vi "蝴蝶图.vi"() -> ()   [LabVIEW 2023]
panel:
  out "XY Graph":cluster{"Y":dbl[], "Y":dbl[]}[](graph)
  out "return value":dbl[][](array[numeric])
  in  "Array 3":dbl[][](array[numeric])
  in  "module path 2":path
  out "error out 2":errorcluster
  out "error out":errorcluster
  in  "module path":path
  out "Array 2":string[](array[string])
  in  "String":string
  in  "Array":string[](array[string])
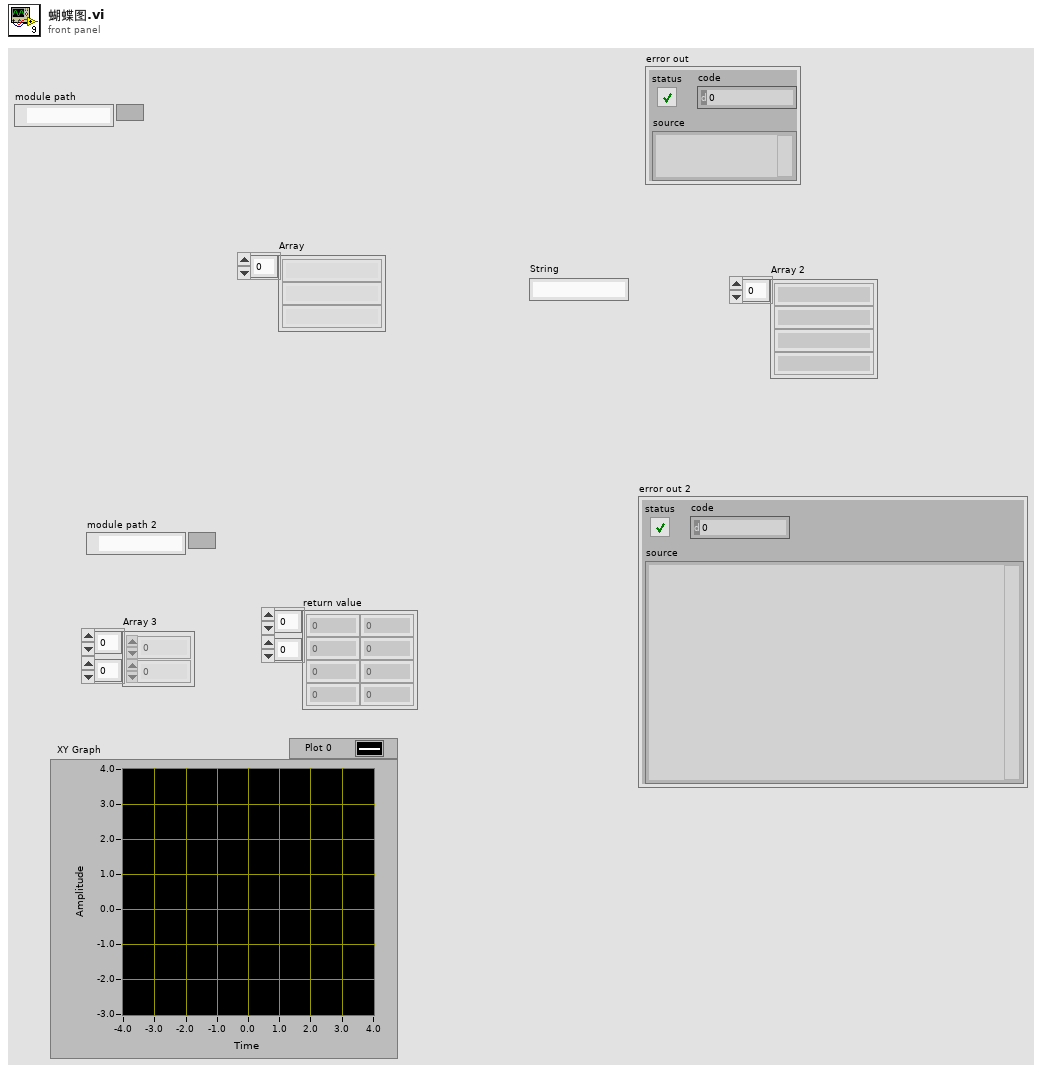
[diagram p1: front panel]
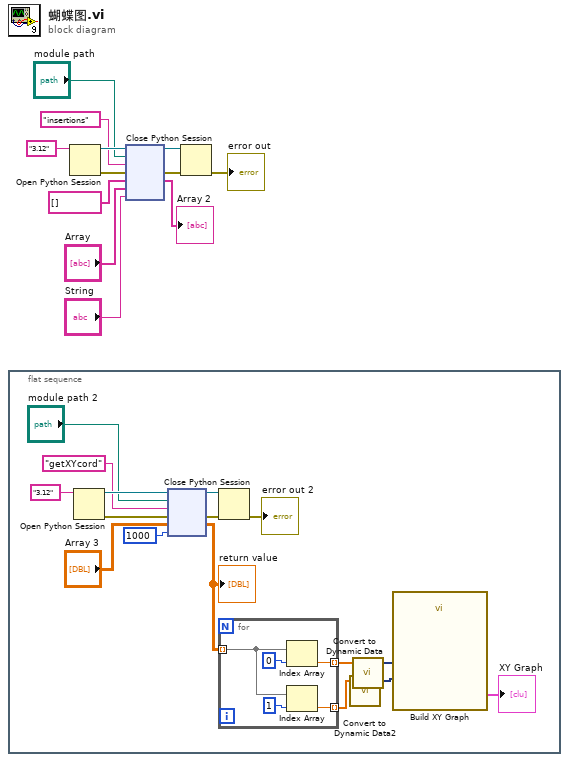
[diagram p0: block diagram]
diagram:
  n1 = flat-sequence {
    frame #0 {
      n2 = Open Python Session(python version="3.12" ("Python version")) -> (session out=w28:refnum<k35>, error out=w26:errorcluster)  [unwired: 2 in]
      n3 = node(w28, "module path 2", "getXYcord" ("function name"), w26, "Array 3", 1000) -> (w27:refnum<k35>, w25:errorcluster, w18:dbl[][])  [unwired: 1 in, 2 out]
      "return value" <- w18
      n4 = Close Python Session(session in=w27, error in=w25) -> (11:→"error out 2":errorcluster)
      n5 = for {
        tunnel: w18 -> [w32] mode=indexing
        tunnel: [w30] -> w16 mode=indexing
        tunnel: [w29] -> w14 mode=indexing
        n6 = Index Array(array=w32, index=0) -> (element=w30:dbl)
        n7 = Index Array(array=w32, index=1) -> (element=w29:dbl)
      }
      n8 = call "Convert to Dynamic Data2"("Array"=w14) -> ("Dynamic Data Type"=w13:dynamicdata)  [unwired: 3 in]
      n9 = call "Convert to Dynamic Data"("Array"=w16) -> ("Dynamic Data Type"=w15:dynamicdata)  [unwired: 3 in]
      n10 = call "Build XY Graph"("Y Input"=w13, "X Input"=w15) -> ("XY Graph"=→"XY Graph":cluster{"X":dbl[], "Y":dbl[]}[])  [unwired: 8 in, 1 out]
    }
  }
  n11 = Open Python Session(python version="3.12" ("Python version")) -> (session out=w11:refnum<k35>, error out=w7:errorcluster)  [unwired: 2 in]
  n12 = node(w11, "module path", "insertions" ("function name"), w7, string[] [], "Array", "String") -> (w9:refnum<k35>, w8:errorcluster, →"Array 2":string[])  [unwired: 2 in, 2 out]
  n13 = Close Python Session(session in=w9, error in=w8) -> (11:→"error out":errorcluster)
